vi "array -- linear regression 3D -- V2.vi"(7 "action":T3, 9 "fit map IN":map{T1, dbl}(c390), 11 "xyzw IN":T2={"x"=[0.0, 0.0, 0.0, -1.0, -1.0, -1.0, 1.0, 1.0, 1.0], "y"=[-1.0, 0.0, 1.0, -1.0, 0.0, 1.0, -1.0, 0.0, 1.0], "z"=[1.0, 0.0, 1.0, 4.0, 1.0, 0.0, 0.0, 1.0, 4.0], "w"=[-1.0, 0.0, 1.0, -1.0, 0.0, 1.0, -1.0, 0.0, 1.0]}) -> (1 "fit map out":map{T1, dbl}(c390), 3 "xyz OUT":T2={"x"=[0.0, 0.0, 0.0, -1.0, -1.0, -1.0, 1.0, 1.0, 1.0], "y"=[-1.0, 0.0, 1.0, -1.0, 0.0, 1.0, -1.0, 0.0, 1.0], "z"=[1.0, 0.0, 1.0, 4.0, 1.0, 0.0, 0.0, 1.0, 4.0], "w"=[-1.0, 0.0, 1.0, -1.0, 0.0, 1.0, -1.0, 0.0, 1.0]})   [LabVIEW 2021]
uses:
  array -- fit control .ctl
  array -- bilinear regression 2D.ctl
  <vilib>/Analysis/baseanly.llb/Matrix Type of Inverse Matrix.ctl
  <vilib>/Analysis/baseanly.llb/Real A x B.vi
  <vilib>/Analysis/Matrix/Numeric/Conversions/Array To Matrix - RA2.vi
  <vilib>/Analysis/baseanly.llb/Real Inverse Matrix.vi
  <vilib>/Analysis/Matrix/Numeric/Conversions/Matrix To Array - RM.vi
  <vilib>/Analysis/NI_AALBase.lvlib
  <vilib>/Analysis/Matrix/NI_Matrix.lvlib
panel:
  out "fit out":dbl[](array[numeric])=[1.9, 2.6, 3.3, 1.0, 2.7, 3.9]
  out "w":dbl[](array[numeric])=[-1.0, 0.0, 1.0, -1.0, 0.0, 1.0, -1.0, 0.0, 1.0]
  out "y":dbl[](array[numeric])=[-1.0, 0.0, 1.0, -1.0, 0.0, 1.0, -1.0, 0.0, 1.0]
  out "fit  IN":dbl[](array[numeric])=[1.9, 2.6, 3.3, 1.0, 2.7, 3.9]
  out "z":dbl[](array[numeric])=[1.0, 0.0, 1.0, 4.0, 1.0, 0.0, 0.0, 1.0, 4.0]
  out "x":dbl[](array[numeric])=[0.0, 0.0, 0.0, -1.0, -1.0, -1.0, 1.0, 1.0, 1.0]
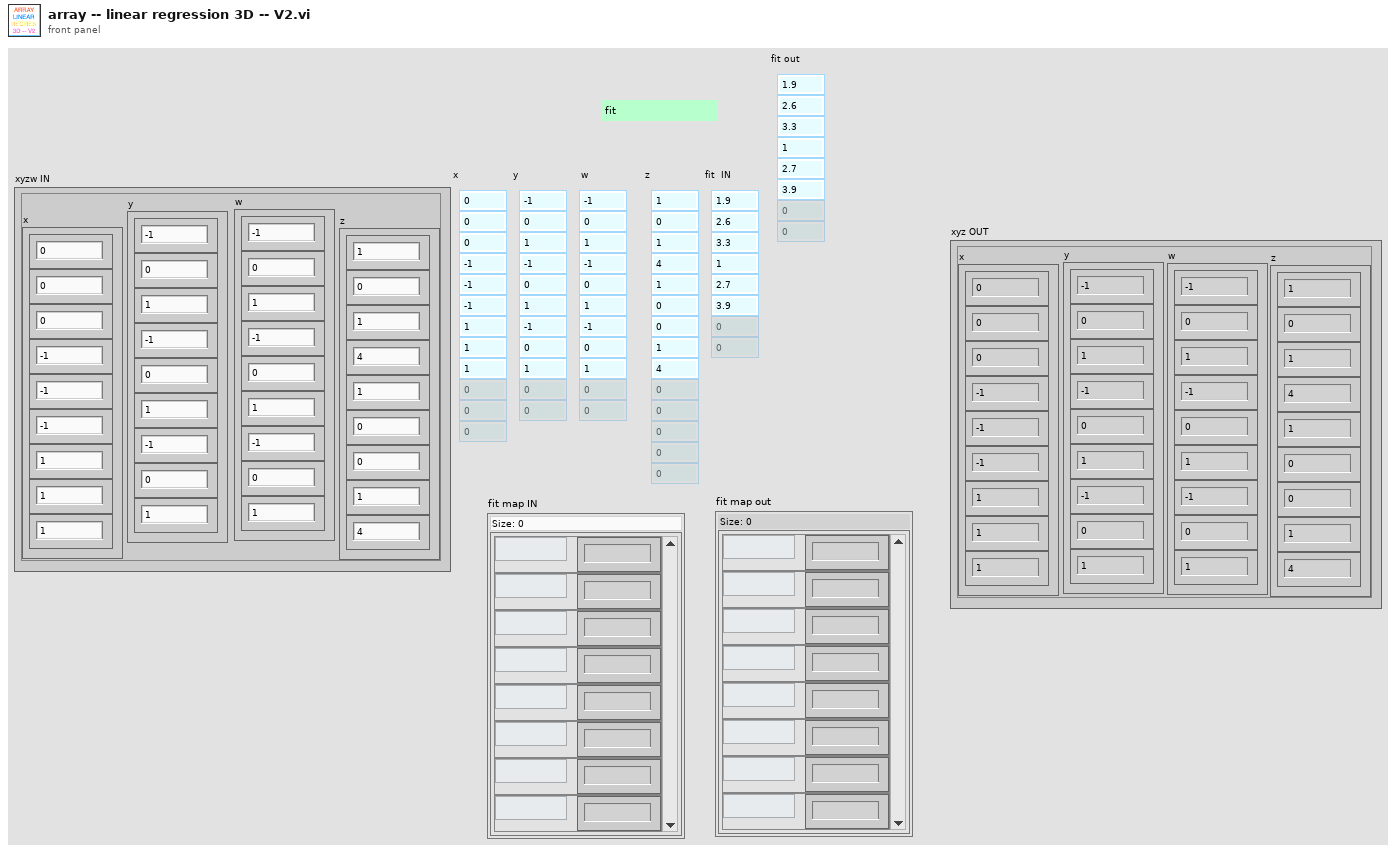
[diagram p1: front panel]
types:
  T1 = typedef "array -- bilinear regression 2D.ctl" = enum16{"1", "x", "y", "xx", "xy", "yy", "xxy", "xyy", "yyy", "xxx", "xxyy", "xyyy", "xxxy", "yyyy", "xxxx", "xxz", "xyz", "yyz", "xz", "yz", "z", "wwz", "ywz", "xwz", "xxxw", "xxyw", "xyyw", "yyyw", "xxww", "xyww", "yyww", "xwww", "ywww", "wwww", "ww", "xw", "yw", "w", "wz"}
  T2 = cluster{"x":dbl[], "y":dbl[], "z":dbl[], "w":dbl[]}
  T3 = typedef "array -- fit control .ctl" = enum16{"fit", "calc", "check", "init"}
  T4 = typedef "NI_AALBase.lvlib/Matrix Type of Inverse Matrix.ctl" = enum32{"General", "Positive Definite", "Lower Triangular", "Upper Triangular"}
  T5 = typedef "NI_Matrix.lvlib/RealMatrix.ctl" = dbl[][]
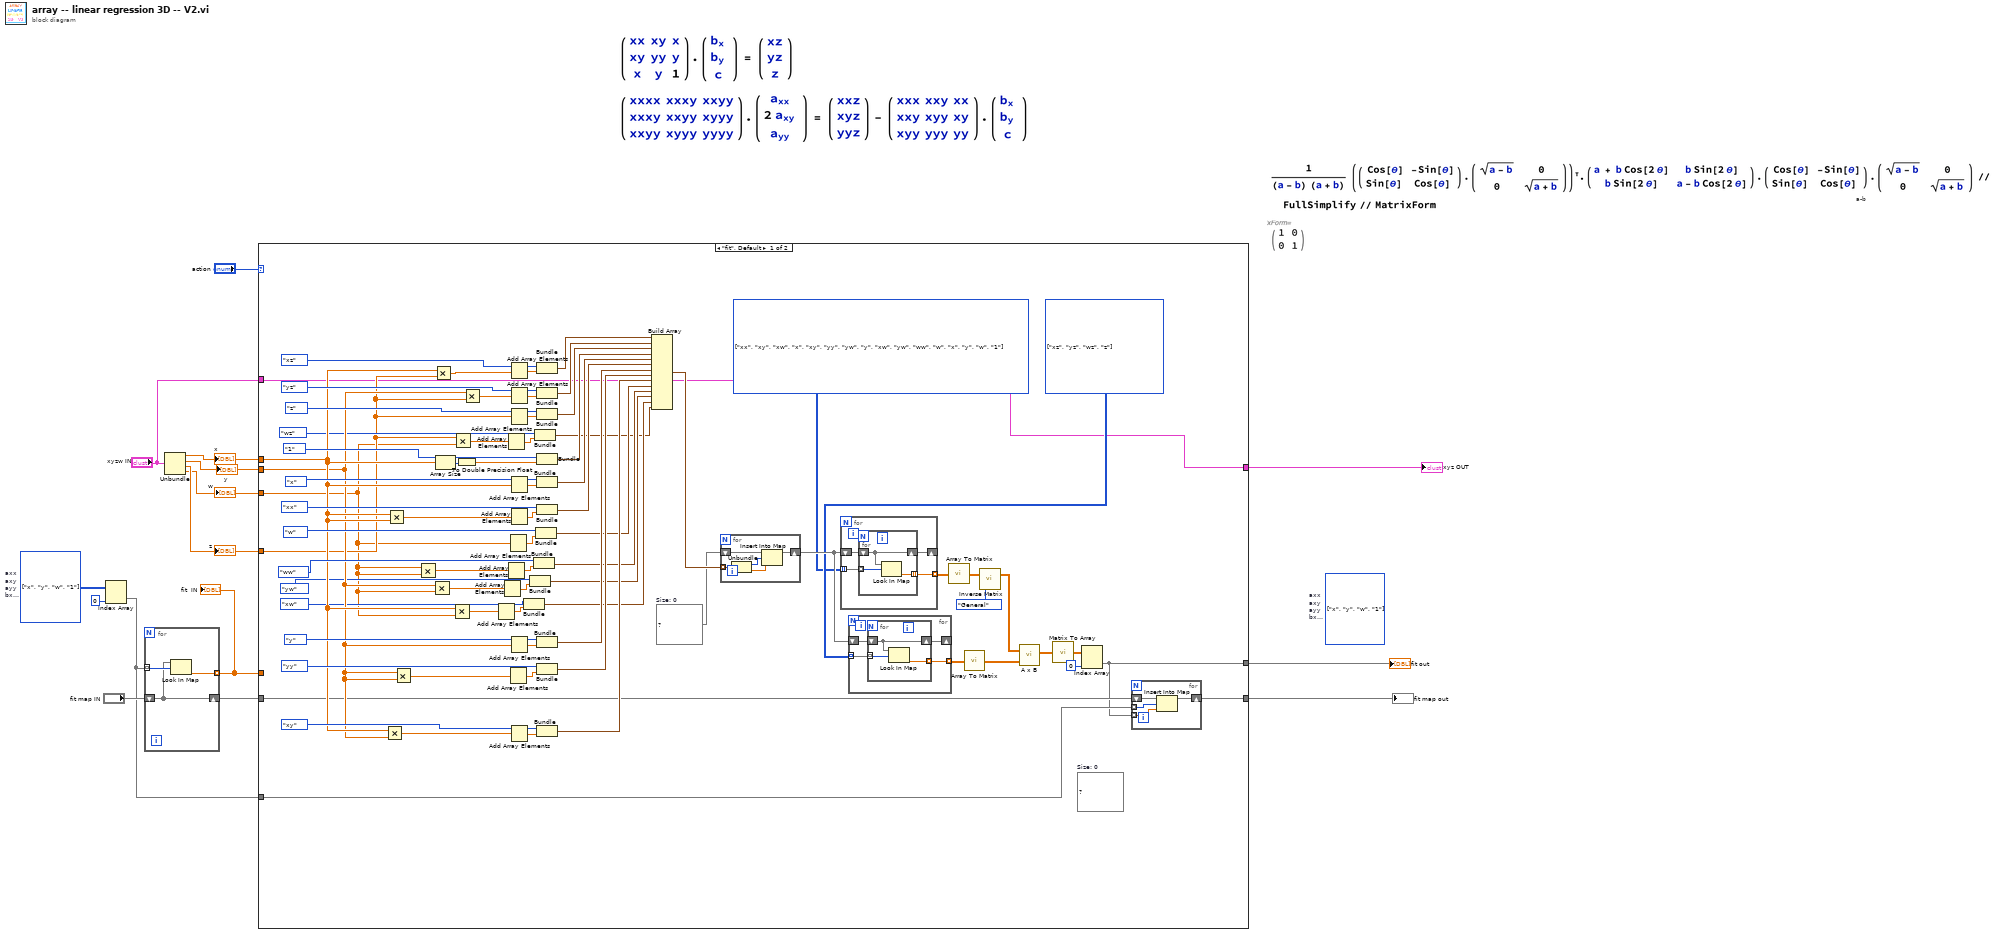
[diagram p0: block diagram]
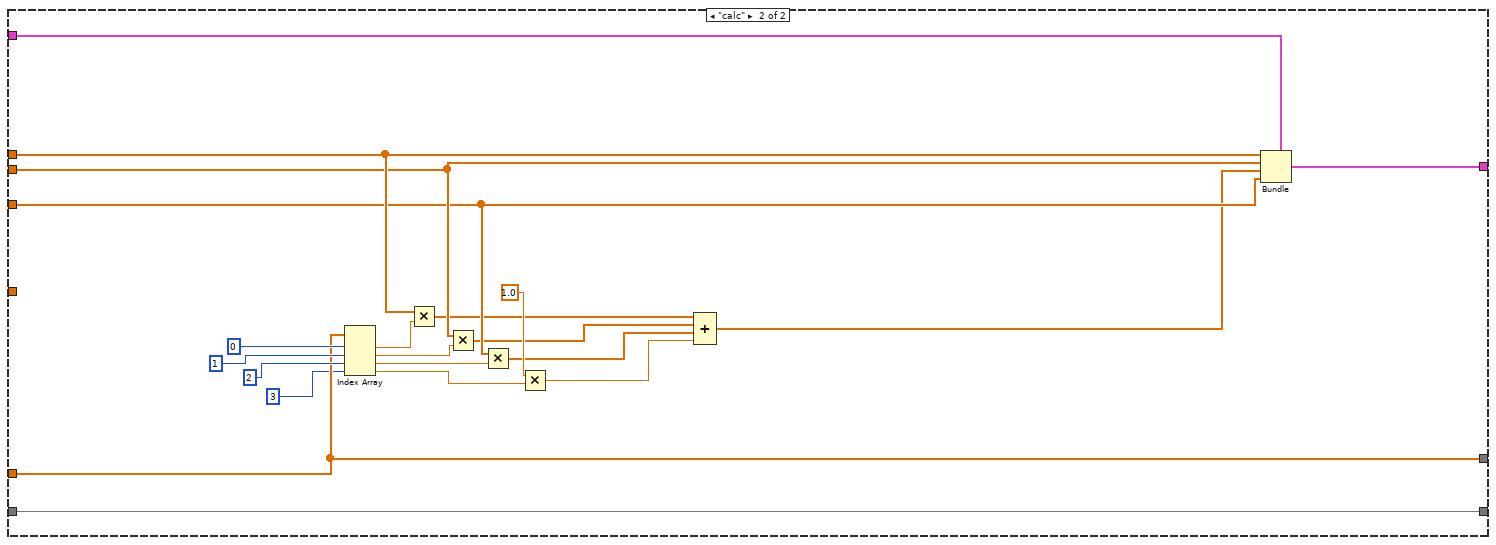
[diagram p2: hidden frame]
diagram:
  (unwired) T1[][] [[enum."x"], [enum."y"], [enum."w"], [enum."1"]] items=["1", "x", "y", "xx", "xy", "yy", "xxy", "xyy", "yyy", "xxx", "xxyy", "xyyy", "xxxy", "yyyy", "xxxx", "xxz", "xyz", "yyz", "xz", "yz", "z", "wwz", "ywz", "xwz", "xxxw", "xxyw", "xyyw", "yyyw", "xxww", "xyww", "yyww", "xwww", "ywww", "wwww", "ww", "xw", "yw", "w", "wz"]  # axx axy ayy bx by c
  w8 = T1[][] [[enum."x"], [enum."y"], [enum."w"], [enum."1"]] items=["1", "x", "y", "xx", "xy", "yy", "xxy", "xyy", "yyy", "xxx", "xxyy", "xyyy", "xxxy", "yyyy", "xxxx", "xxz", "xyz", "yyz", "xz", "yz", "z", "wwz", "ywz", "xwz", "xxxw", "xxyw", "xyyw", "yyyw", "xxww", "xyww", "yyww", "xwww", "ywww", "wwww", "ww", "xw", "yw", "w", "wz"]  # axx axy ayy bx by c
  # "a-b"
  n1 = Index Array(array=w8, index (col)=0 ("disabled index (col)")) -> (element=w5:T1[])  [unwired: 1 in]
  n2 = for {
    tunnel: w5 -> [w18] mode=indexing
    shift-right: [w17] -> w6
    shift-left: "fit map IN" -> [w17]
    tunnel: [w16] -> w9 mode=indexing
    n3 = Look In Map(map=w17, key=w18) -> (value=w16:dbl)  [unwired: 1 in, 1 out]
  }
  "fit  IN" <- w9
  n4 = Unbundle("xyzw IN") -> ("x"=w14:dbl[], "y"=w13:dbl[], "z"=w12:dbl[], "w"=w7:dbl[])
  "x" <- w14
  "z" <- w12
  "y" <- w13
  "w" <- w7
  n5 = case shown="\"fit\", Default" "action" {
    tunnel: w12 -> [w33 _]
    tunnel: w14 -> [w38 w128]
    tunnel: [w20 w134] -> w3
    tunnel: w9 -> [_ w134]
    tunnel: w13 -> [w37 w127]
    tunnel: w7 -> [w25 w126]
    tunnel: w6 -> [w21 w118]
    tunnel: w5 -> [w23 _]
    tunnel: [w22 w118] -> w4
    tunnel: "xyzw IN" -> [w19 w120]
    tunnel: [w19 w117] -> w1
    frame "fit", Default {
      (unwired) map{T1, dbl} {}  # Size: 0
      w51 = T1[][] [[enum."xz"], [enum."yz"], [enum."wz"], [enum."z"]] items=["1", "x", "y", "xx", "xy", "yy", "xxy", "xyy", "yyy", "xxx", "xxyy", "xyyy", "xxxy", "yyyy", "xxxx", "xxz", "xyz", "yyz", "xz", "yz", "z", "wwz", "ywz", "xwz", "xxxw", "xxyw", "xyyw", "yyyw", "xxww", "xyww", "yyww", "xwww", "ywww", "wwww", "ww", "xw", "yw", "w", "wz"]
      w50 = T1[][] [[enum."xx", enum."xy", enum."xw", enum."x"], [enum."xy", enum."yy", enum."yw", enum."y"], [enum."xw", enum."yw", enum."ww", enum."w"], [enum."x", enum."y", enum."w", enum."1"]] items=["1", "x", "y", "xx", "xy", "yy", "xxy", "xyy", "yyy", "xxx", "xxyy", "xyyy", "xxxy", "yyyy", "xxxx", "xxz", "xyz", "yyz", "xz", "yz", "z", "wwz", "ywz", "xwz", "xxxw", "xxyw", "xyyw", "yyyw", "xxww", "xyww", "yyww", "xwww", "ywww", "wwww", "ww", "xw", "yw", "w", "wz"]
      w24 = map{T1, dbl} {}  # Size: 0
      n6 = Multiply(x=w38, y=w37) -> (x*y=w49:dbl[])
      n7 = Multiply(x=w38, y=w38) -> (x*y=w87:dbl[])
      n8 = Multiply(x=w37, y=w37) -> (x*y=w88:dbl[])
      n9 = Multiply(x=w25, y=w25) -> (x*y=w46:dbl[])
      n10 = Multiply(x=w37, y=w25) -> (x*y=w40:dbl[])
      n11 = Multiply(x=w38, y=w33) -> (x*y=w86:dbl[])
      n12 = Array Size(array=w38) -> (size(s)=w76:i32)
      n13 = Multiply(x=w38, y=w25) -> (x*y=w39:dbl[])
      n14 = Multiply(x=w33, y=w25) -> (x*y=w35:dbl[])
      n15 = To Double Precision Float(number=w76) -> (double precision float=w64:dbl)
      n16 = Multiply(x=w37, y=w33) -> (x*y=w89:dbl[])
      n17 = Add Array Elements(numeric array=w39) -> (sum=w43:dbl)
      n18 = Add Array Elements(numeric array=w40) -> (sum=w44:dbl)
      n19 = Add Array Elements(numeric array=w35) -> (sum=w36:dbl)
      n20 = Add Array Elements(numeric array=w46) -> (sum=w47:dbl)
      n21 = Add Array Elements(numeric array=w88) -> (sum=w83:dbl)
      n22 = Add Array Elements(numeric array=w25) -> (sum=w42:dbl)
      n23 = Add Array Elements(numeric array=w86) -> (sum=w73:dbl)
      n24 = Add Array Elements(numeric array=w89) -> (sum=w71:dbl)
      n25 = Add Array Elements(numeric array=w33) -> (sum=w69:dbl)
      n26 = Add Array Elements(numeric array=w38) -> (sum=w78:dbl)
      n27 = Add Array Elements(numeric array=w87) -> (sum=w79:dbl)
      n28 = Add Array Elements(numeric array=w37) -> (sum=w82:dbl)
      n29 = Add Array Elements(numeric array=w49) -> (sum=w60:dbl)
      n30 = Bundle(array_--_bilinear_regression_2D."xw", "Numeric"=w43) -> (w27:cluster{T1, "Numeric":dbl})  [unwired: 1 in]
      n31 = Bundle(array_--_bilinear_regression_2D."yw", "Numeric"=w44) -> (w30:cluster{T1, "Numeric":dbl})  [unwired: 1 in]
      n32 = Bundle(array_--_bilinear_regression_2D."ww", "Numeric"=w47) -> (w31:cluster{T1, "Numeric":dbl})  [unwired: 1 in]
      n33 = Bundle(array_--_bilinear_regression_2D."wz", "Numeric"=w36) -> (w26:cluster{T1, "Numeric":dbl})  [unwired: 1 in]
      n34 = Bundle(array_--_bilinear_regression_2D."w", "Numeric"=w42) -> (w32:cluster{T1, "Numeric":dbl})  [unwired: 1 in]
      n35 = Bundle(array_--_bilinear_regression_2D."xz", "Numeric"=w73) -> (w68:cluster{T1, "Numeric":dbl})  [unwired: 1 in]
      n36 = Bundle(array_--_bilinear_regression_2D."yz", "Numeric"=w71) -> (w67:cluster{T1, "Numeric":dbl})  [unwired: 1 in]
      n37 = Bundle(array_--_bilinear_regression_2D."z", "Numeric"=w69) -> (w66:cluster{T1, "Numeric":dbl})  [unwired: 1 in]
      n38 = Bundle(array_--_bilinear_regression_2D."1", w64) -> (w65:cluster{T1, dbl})  [unwired: 1 in]
      n39 = Bundle(array_--_bilinear_regression_2D."x", "Numeric"=w78) -> (w63:cluster{T1, "Numeric":dbl})  [unwired: 1 in]
      n40 = Bundle(array_--_bilinear_regression_2D."xx", "Numeric"=w79) -> (w62:cluster{T1, "Numeric":dbl})  [unwired: 1 in]
      n41 = Bundle(array_--_bilinear_regression_2D."y", "Numeric"=w82) -> (w61:cluster{T1, "Numeric":dbl})  [unwired: 1 in]
      n42 = Bundle(array_--_bilinear_regression_2D."yy", "Numeric"=w83) -> (w53:cluster{T1, "Numeric":dbl})  [unwired: 1 in]
      n43 = Bundle(array_--_bilinear_regression_2D."xy", "Numeric"=w60) -> (w48:cluster{T1, "Numeric":dbl})  [unwired: 1 in]
      n44 = Build Array(w68, w67, w66, w65, w63, w62, w61, w53, w48, w32, w31, w30, w27, w26) -> (w59:cluster{T1, "Numeric":dbl}[])
      n45 = for {
        tunnel: w59 -> [w107] mode=indexing
        shift-right: [w108] -> w52
        shift-left: w24 -> [w109]
        n46 = Unbundle(w107) -> (w106:T1, "Numeric"=w105:dbl)
        n47 = Insert Into Map(map in=w109, key=w106, value=w105) -> (map out=w108:map{T1, dbl})  [unwired: 2 out]
      }
      n48 = for {
        tunnel: w50 -> [w113] mode=indexing
        shift-right: [w111] -> _
        shift-left: w52 -> [w112]
        tunnel: [w110] -> w57 mode=indexing
        n49 = for {
          tunnel: w113 -> [w115] mode=indexing
          shift-right: [w116] -> w111
          shift-left: w112 -> [w116]
          tunnel: [w114] -> w110 mode=indexing
          n50 = Look In Map(map=w116, key=w115) -> (value=w114:dbl)  [unwired: 1 in, 1 out]
        }
      }
      n51 = for {
        shift-right: [w100] -> _
        shift-left: w52 -> [w101]
        tunnel: w51 -> [w99] mode=indexing
        tunnel: [w98] -> w56 mode=indexing
        n52 = for {
          shift-right: [w104] -> w100
          shift-left: w101 -> [w104]
          tunnel: w99 -> [w103] mode=indexing
          tunnel: [w102] -> w98 mode=indexing
          n53 = Look In Map(map=w104, key=w103) -> (value=w102:dbl)  [unwired: 1 in, 1 out]
        }
      }
      n54 = call-poly <vilib>:"Array To Matrix.vi"("Real 2D Array"=w57) -> ("Real Matrix"=w54:T5)
      n55 = call-poly <vilib>:"Array To Matrix.vi"("Real 2D Array"=w56) -> ("Real Matrix"=w55:T5)
      n56 = call-poly <vilib>:"Inverse Matrix.vi"("matrix type"=Matrix_Type_of_Inverse_Matrix."General", "Input Matrix"=w54) -> ("Inverse Matrix"=w93:T5)  [unwired: 1 out]
      n57 = call-poly <vilib>:"A x B.vi"("B"=w55, "A"=w93) -> ("A x B"=w92:T5)  [unwired: 1 out]
      n58 = call-poly <vilib>:"Matrix To Array.vi"("Real Matrix"=w92) -> ("Real 2D Array"=w91:dbl[][])
      n59 = Index Array(array=w91, index (col)=0 ("disabled index (col)")) -> (element=w20:dbl[])  [unwired: 1 in]
      n60 = for {
        shift-right: [w96] -> w22
        shift-left: w21 -> [w97]
        tunnel: w23 -> [w95] mode=indexing
        tunnel: w20 -> [w94] mode=indexing
        n61 = Insert Into Map(map in=w97, key=w95, value=w94) -> (map out=w96:map{T1, dbl})  [unwired: 2 out]
      }
    }
    frame "calc" {
      n62 = Index Array(array=w134, index #1=0 ("index"), index #2=1 ("index"), index #3=2 ("index"), index #4=3 ("index")) -> (element #1=w132:dbl, element #2=w131:dbl, element #3=w130:dbl, element #4=w129:dbl)
      n63 = Multiply(x=w128, y=w132) -> (x*y=w124:dbl[])
      n64 = Multiply(x=w127, y=w131) -> (x*y=w123:dbl[])
      n65 = Multiply(x=w126, y=w130) -> (x*y=w122:dbl[])
      n66 = Multiply(x=1.0, y=w129) -> (x*y=w121:dbl)
      n67 = Compound Arithmetic op=ADD(w124, w123, w122, w121) -> (w119:dbl[])
      n68 = Bundle(cluster=w120, "x"=w128, "y"=w127, "z"=w119, "w"=w126) -> (w117:T2)
    }
  }
  "fit map out" <- w4
  "xyz OUT" <- w1
  "fit out" <- w3
